vi "GEN_WriteStatus.vi"(7 "Input String":string, 8 "error in (no error)":errorcluster, 10 "Config_Cluster":T1={"General"={"Config.ini"=path "", "Default Logging Path"=path ""}, "Hardware"={"AHC VISA COM"="", "Measure Rate (1/s)"=0, "Global T VAR"="", "Global B VAR"="", "Average"=4, "Bias"=0, "Cable"={"Length"=0.0, "Resistance"=0.0, "Inductance"=0.0, "Capacitance"=0.0}, "Tracking"=0, "Voltage"=0.0}, "Operation"={"Operation Mode"=enum."Idle-Off", "Status"="", "NewLog?"=FALSE}}, 11 "Status Ref":refnum<vi>) -> (0 "error out":errorcluster, 2 "Config_Cluster Out":T1={"General"={"Config.ini"=path "", "Default Logging Path"=path ""}, "Hardware"={"AHC VISA COM"="", "Measure Rate (1/s)"=0, "Global T VAR"="", "Global B VAR"="", "Average"=4, "Bias"=0, "Cable"={"Length"=0.0, "Resistance"=0.0, "Inductance"=0.0, "Capacitance"=0.0}, "Tracking"=0, "Voltage"=0.0}, "Operation"={"Operation Mode"=enum."Idle-Off", "Status"="", "NewLog?"=FALSE}})   [LabVIEW 2021]
uses:
  Config_Cluster.ctl
  Mode_Enum.ctl
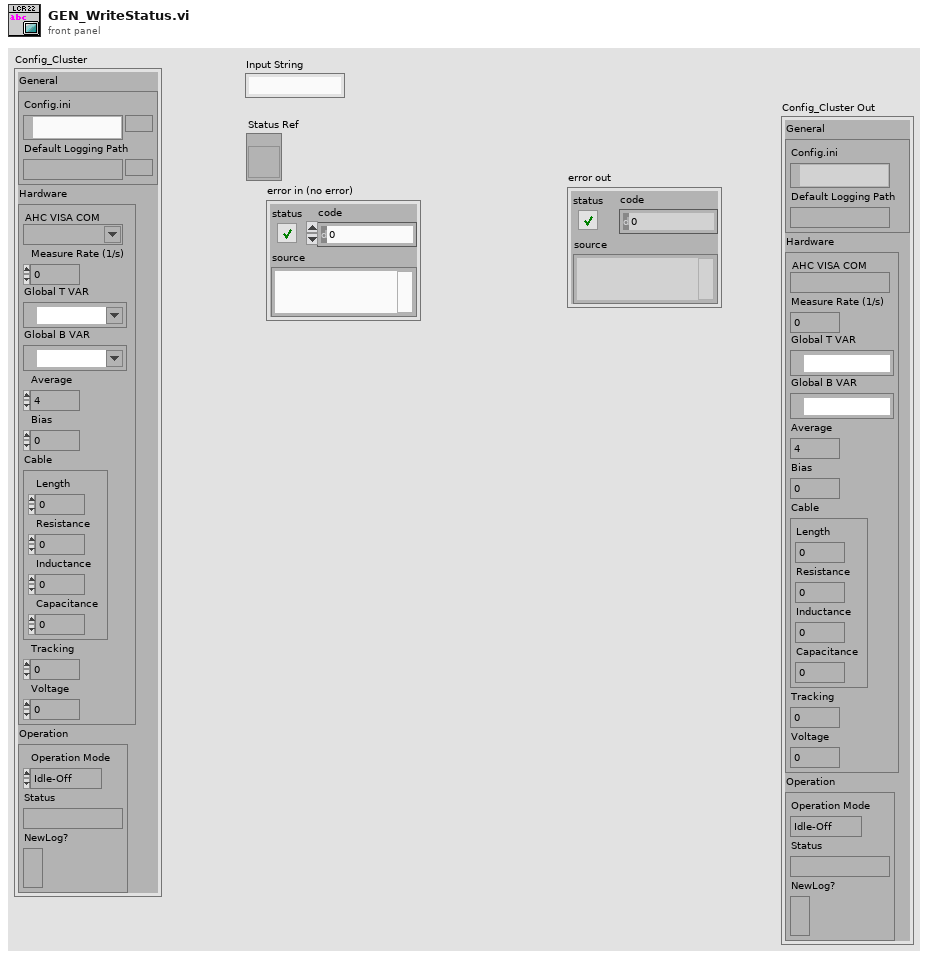
[diagram p1: front panel]
types:
  T1 = typedef "Config_Cluster.ctl" = cluster{"General":cluster{"Config.ini":path, "Default Logging Path":path}, "Hardware":cluster{"AHC VISA COM":refnum<visa-resource-name>, "Measure Rate (1/s)":i32, "Global T VAR":refnum<k21>, "Global B VAR":refnum<k21>, "Average":u8, "Bias":u8, "Cable":cluster{"Length":dbl, "Resistance":dbl, "Inductance":dbl, "Capacitance":dbl}, "Tracking":u8, "Voltage":dbl}, "Operation":cluster{"Operation Mode":T2, "Status":string, "NewLog?":bool}}
  T2 = typedef "Mode_Enum.ctl" = enum16{"Logging", "Idle-Off", "Idle"}
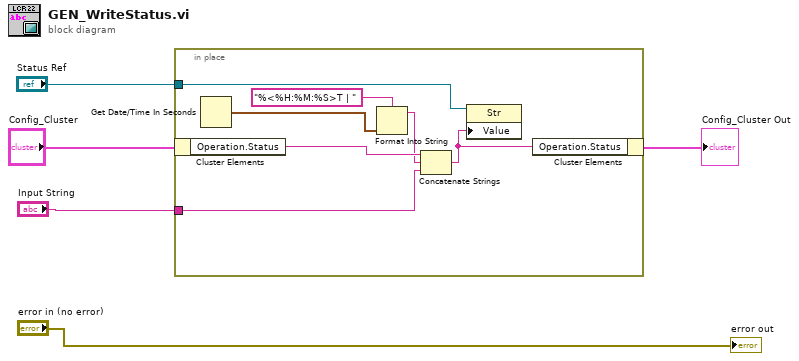
[diagram p0: block diagram]
diagram:
  n1 = in-place {
    in-place-border: "Input String" -> [w7]
    in-place-border: "Status Ref" -> [w11]
    n2 = in-place-cluster #1("Config_Cluster") -> ("Operation.Status"=w12:string)
    n3 = Get Date/Time In Seconds() -> (seconds since 1Jan1904=w9:timestamp)
    n4 = Format Into String(format string="%<%H:%M:%S>T | ", w9) -> (resulting string=w6:string)  [unwired: 2 in, 1 out]
    n5 = Concatenate Strings(w12, w6, w7) -> (w10:string)
    n6 = property class="Str"(reference=w11, "Value"=w10) -> ()  [unwired: 1 in, 2 out]
    n7 = in-place-cluster #1("Operation.Status"=w10) -> (→"Config_Cluster Out":T1)
  }
  "error out" <- "error in (no error)"
